vi "Omron TCP FINS-Read Data(I16 Element).vi"(8 "error in":errorcluster, 10 "Read Setting(I16 Element)":T1={"I/O Memory Address"=130, "Data Address"=0} {"I/O Memory Address" items=["DM"=130, "CIO"=176, "WR"=177, "HR"=178, "AR"=179, "TIM"=137, "EM"=152]}, 11 "Buffer Data In":T2) -> (0 "error out":errorcluster, 2 "Data":i16, 3 "Buffer Data Out":T2)   [LabVIEW 2016]
uses:
  Data Def/Omron TCP FINS-Buffer Data.ctl
  Data Def/Omron TCP FINS-Command Code.ctl
  Data Def/Omron TCP FINS-FINS Command Frame.ctl
  Data Def/Omron TCP FINS-Memory Area Read Data.ctl
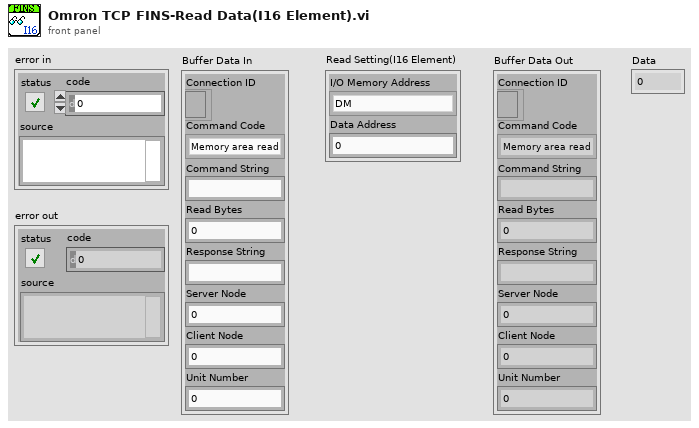
[diagram p1: front panel]
types:
  T1 = cluster{"I/O Memory Address":u8, "Data Address":u16}
  T2 = typedef "Omron TCP FINS-Buffer Data.ctl" = cluster{"Connection ID":refnum<k5>, "Command Code":T3, "Command String":string, "Read Bytes":i32, "Response String":string, "Server Node":u8, "Client Node":u8, "Unit Number":u8}
  T3 = typedef "Omron TCP FINS-Command Code.ctl" = enum16{"Memory area read", "Memory area write"}
  T4 = typedef "Omron TCP FINS-Memory Area Read Data.ctl" = cluster{"I/O Memory Address":u8, "Beginning Address":u16, "No. Of Items":u16}
  T5 = typedef "Omron TCP FINS-FINS Command Frame.ctl" = cluster{"Command Code":T3, "Command Data":variant}
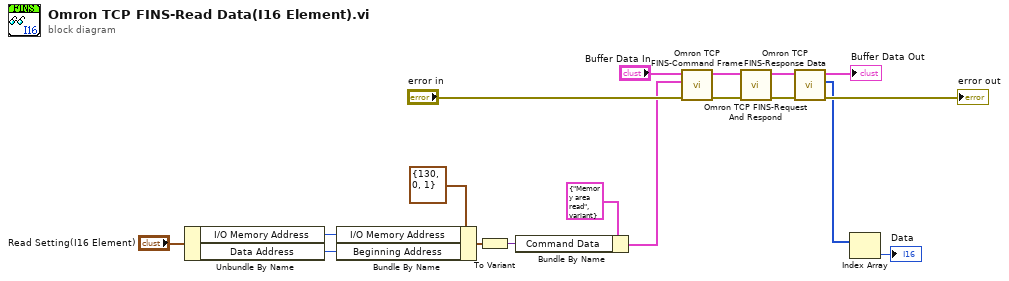
[diagram p0: block diagram]
diagram:
  n1 = Unbundle By Name("Read Setting(I16 Element)") -> ("I/O Memory Address"=w4:u8, "Data Address"=w3:u16)
  n2 = Bundle By Name(cluster=T4 {"I/O Memory Address"=130, "Beginning Address"=0, "No. Of Items"=1} ("Memory Area Read Data"), "I/O Memory Address"=w4, "Beginning Address"=w3) -> (w7:T4)
  n3 = To Variant(anything=w7) -> (Variant=w16:variant)
  n4 = Bundle By Name(cluster=T5 {"Command Code"=enum."Memory area read", "Command Data"=variant} ("FINS Command Frame"), "Command Data"=w16) -> (w14:T5)
  n5 = call "Omron TCP FINS-Command Frame.vi"("error in"="error in", "FINS Command Frame"=w14, "Buffer Data In"="Buffer Data In") -> ("error out"=w12:errorcluster, "Buffer Data Out"=w13:T2)  [unwired: 7 in]
  n6 = call "Omron TCP FINS-Request And Respond.vi"("error in"=w12, "Buffer Data In"=w13) -> ("error out"=w10:errorcluster, "Buffer Data Out"=w11:T2)  [unwired: 8 in]
  n7 = call "Omron TCP FINS-Response Data.vi"("error in"=w10, "Buffer Data In"=w11) -> ("error out"=→"error out":errorcluster, "Data"=w2:i16[], "Buffer Data Out"=→"Buffer Data Out":T2)  [unwired: 7 in]
  n8 = Index Array(array=w2) -> (element=→"Data":i16)  [unwired: 1 in]
